vi "remove current DC component.vi"(11 "Acquired Data":T1) -> (3 "Acquired Data out":T1)   [LabVIEW 2019, in "Main.lvclass"]
doc: "Developed by Kevin Thompson\nkevin@thompsonengineering.net\n\nCopyright 2020\nThompson Engineering, LLC"
uses:
  Main.lvclass
  DataTypes/raw data variables.ctl
  <vilib>/Analysis/NI_AALPro.lvlib
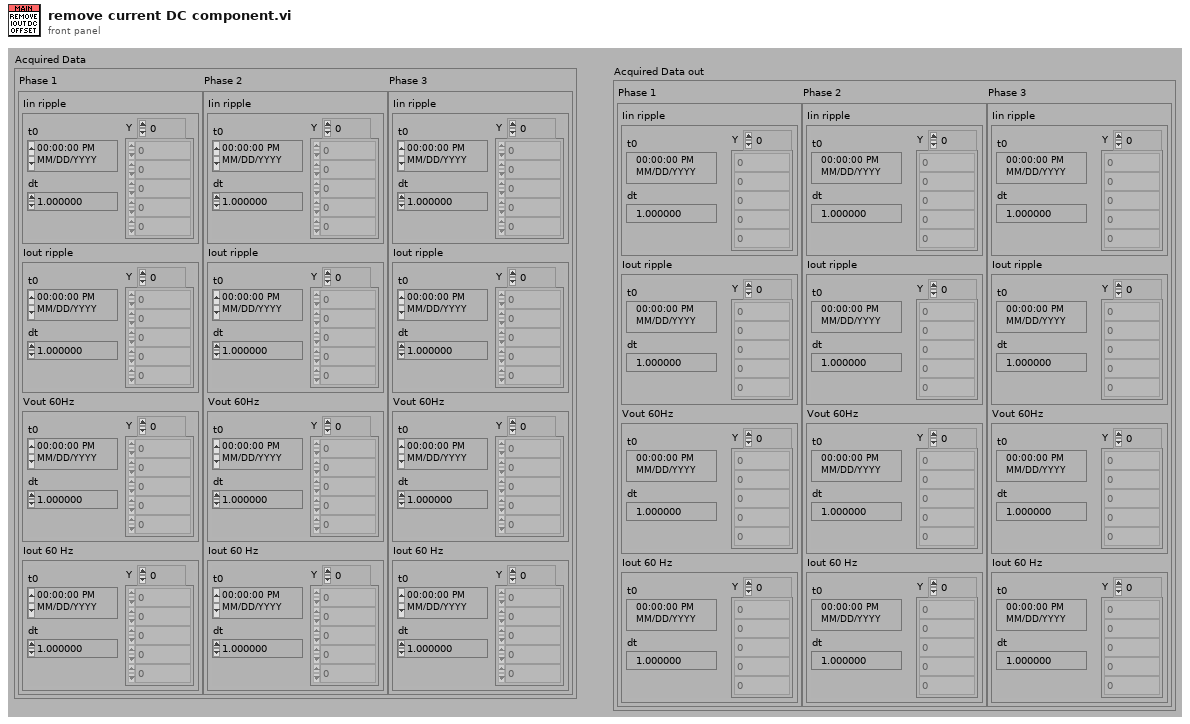
[diagram p1: front panel]
types:
  T1 = typedef "Main.lvclass/raw data variables.ctl" = cluster{"Phase 1":cluster{"Iin ripple":waveform(dbl), "Iout ripple":waveform(dbl), "Vout 60Hz":waveform(dbl), "Iout 60 Hz":waveform(dbl)}, "Phase 2":cluster{"Iin ripple":waveform(dbl), "Iout ripple":waveform(dbl), "Vout 60Hz":waveform(dbl), "Iout 60 Hz":waveform(dbl)}, "Phase 3":cluster{"Iin ripple":waveform(dbl), "Iout ripple":waveform(dbl), "Vout 60Hz":waveform(dbl), "Iout 60 Hz":waveform(dbl)}}
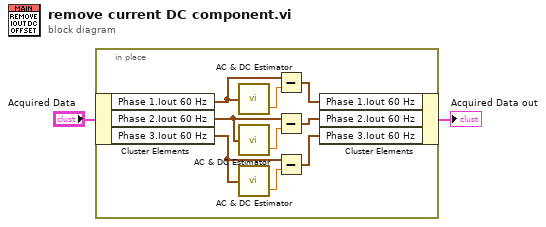
[diagram p0: block diagram]
diagram:
  n1 = in-place {
    n2 = in-place-cluster #1("Acquired Data") -> ("Phase 1.Iout 60 Hz"=w11:waveform(dbl), "Phase 2.Iout 60 Hz"=w8:waveform(dbl), "Phase 3.Iout 60 Hz"=w5:waveform(dbl))
    n3 = call <vilib>:"AC & DC Estimator.vi"("Signal (V)"=w11) -> ("DC estimate (V)"=w10:dbl)  [unwired: 1 out]
    n4 = call <vilib>:"AC & DC Estimator.vi"("Signal (V)"=w8) -> ("DC estimate (V)"=w7:dbl)  [unwired: 1 out]
    n5 = call <vilib>:"AC & DC Estimator.vi"("Signal (V)"=w5) -> ("DC estimate (V)"=w4:dbl)  [unwired: 1 out]
    n6 = Subtract(x=w11, y=w10) -> (x-y=w9:waveform(dbl))
    n7 = Subtract(x=w8, y=w7) -> (x-y=w6:waveform(dbl))
    n8 = Subtract(x=w5, y=w4) -> (x-y=w3:waveform(dbl))
    n9 = in-place-cluster #1("Phase 1.Iout 60 Hz"=w9, "Phase 2.Iout 60 Hz"=w6, "Phase 3.Iout 60 Hz"=w3) -> (→"Acquired Data out":T1)
  }
